vi "CSV Series Reader Tester.vi"() -> ()   [LabVIEW 2018, in "CSV Series Read.lvlib"]
uses:
  CSV Series Read.lvlib
  Data Series.ctl
panel:
  in  "Filenames":string[](array[string])=["e3series.csv", "e6series.csv", "e12series.csv", "e24series.csv", "e48series.csv", "e96series.csv", "e192series.csv"]
  out "Data Series":T1
  out "error out":errorcluster
  in  "error in":errorcluster
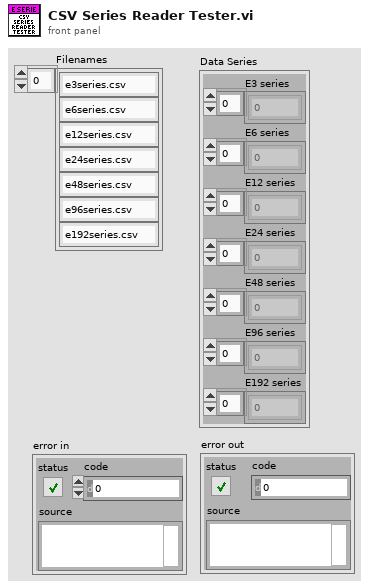
[diagram p1: front panel]
types:
  T1 = typedef "CSV Series Read.lvlib/Data Series.ctl" = cluster{"E3 series":u16[], "E6 series":u16[], "E12 series":u16[], "E24 series":u16[], "E48 series":u16[], "E96 series":u16[], "E192 series":u16[]}
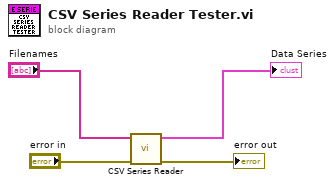
[diagram p0: block diagram]
diagram:
  n1 = call "CSV Series Reader.vi"("error in"="error in", "Filenames"="Filenames") -> ("error out"=→"error out":errorcluster, "Data Series"=→"Data Series":T1)  [unwired: 8 in]
